vi "SaveLogEntry.vi"(8 "error in (no error)":errorcluster, 11 "Logger in":refnum<class "Logger.lvclass">) -> (0 "error out":errorcluster, 3 "Logger out":refnum<class "Logger.lvclass">)   [LabVIEW 2013, in "Logger.lvclass"]
uses:
  Logger.lvclass
  Logger.lvclass/Logger.ctl
  <vilib>/Utility/file.llb/Write To Spreadsheet File (string).vi
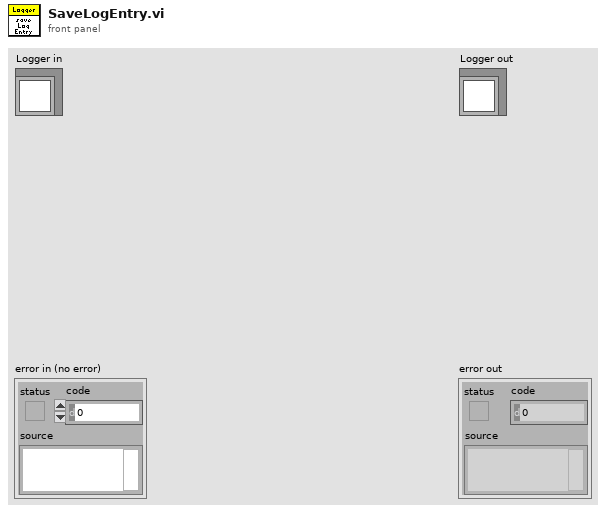
[diagram p1: front panel]
types:
  T1 = typedef "M2AADTTypedefs.lvlib/InputData.ctl" = cluster{"Limit Switches":T2, "SSI Encoder":i32, "Force Measured":T3, "Distance Data":T4, "Thermocouple Data":T5, "Stiffness Data":T6}
  T2 = typedef "ILCCommon.lvlib/ILCTypedefs.lvlib/LimitSwitches.ctl" = cluster{"1":bool, "2":bool}
  T3 = typedef "M2AADTTypedefs.lvlib/ForceDemand.ctl" = dbl[unit]
  T4 = typedef "M2AADTTypedefs.lvlib/Distance Data.ctl" = cluster{"Distance Measured 1":dbl[unit], "Distance Measured 2":dbl[unit]}
  T5 = typedef "M2AADTTypedefs.lvlib/ThermocoupleData.ctl" = cluster{"Motor Temperature":dbl[unit]}
  T6 = typedef "M2AADTTypedefs.lvlib/StiffnessData.ctl" = cluster{"Constrained Displacement":dbl[unit], "Stiffness":dbl[unit]}
  T7 = typedef "M2AADTTypedefs.lvlib/ControllerData.ctl" = cluster{"Force Demand":T3, "Force Error":T3}
  T8 = typedef "M2AADTTypedefs.lvlib/OutputData.ctl" = cluster{"Step & Direction":i16}
  T9 = typedef "M2AADTTypedefs.lvlib/StateSelector.ctl" = enum16{"EndingCycleState", "FaultState", "InteractiveMotionState", "MovingToNewForceState", "OffState", "PausingState", "StandbyState", "StoppedState"}
  T10 = typedef "M2AADTTypedefs.lvlib/TestStatus.ctl" = cluster{"activeCycle":u32, "activeProfileStep":u32}
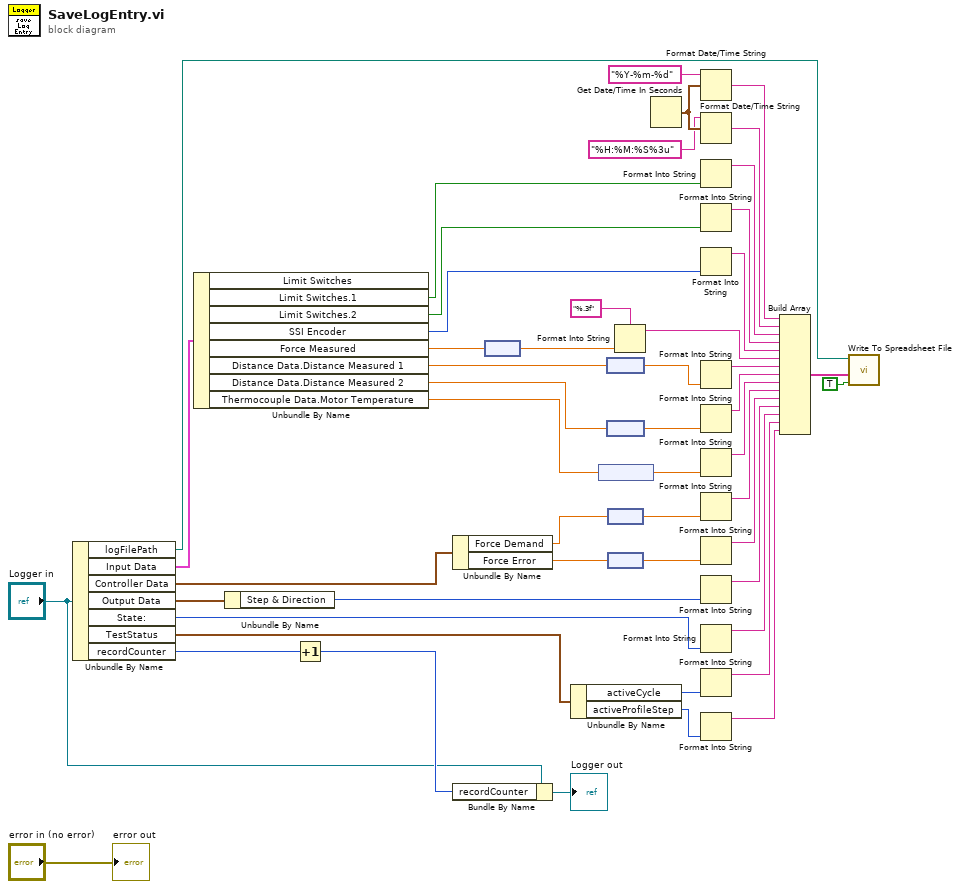
[diagram p0: block diagram]
diagram:
  n1 = Unbundle By Name("Logger in") -> ("logFilePath"=w11:path, "Input Data"=w50:T1, "Controller Data"=w48:T7, "Output Data"=w34:T8, "State:"=w31:T9, "TestStatus"=w16:T10, "recordCounter"=w10:u32)
  n2 = Unbundle By Name(w50) -> ("Limit Switches.1"=w46:bool, "Limit Switches.2"=w44:bool, "SSI Encoder"=w42:i32, "Force Measured"=w28:T3, "Distance Data.Distance Measured 1"=w26:dbl[unit], "Distance Data.Distance Measured 2"=w24:dbl[unit], "Thermocouple Data.Motor Temperature"=w22:dbl[unit])  [unwired: 1 out]
  n3 = Unbundle By Name(w34) -> ("Step & Direction"=w33:i16)
  n4 = Increment(x=w10) -> (x+1=w9:u32)
  n5 = Unbundle By Name(w48) -> ("Force Demand"=w20:T3, "Force Error"=w18:T3)
  n6 = Bundle By Name(cluster="Logger in", "recordCounter"=w9) -> (→"Logger out":refnum<class "Logger.lvclass">)
  n7 = node(w28) -> (w27:dbl)
  n8 = Unbundle By Name(w16) -> ("activeCycle"=w15:u32, "activeProfileStep"=w14:u32)
  n9 = node(w22) -> (w21:dbl)
  n10 = node(w26) -> (w25:dbl)
  n11 = node(w24) -> (w23:dbl)
  n12 = node(w20) -> (w19:dbl)
  n13 = node(w18) -> (w17:dbl)
  n14 = Format Into String(format string="%.3f", w27) -> (resulting string=w40:string)  [unwired: 2 in, 1 out]
  n15 = Get Date/Time In Seconds() -> (seconds since 1Jan1904=w6:timestamp)
  n16 = Format Date/Time String(time format string (%c)="%Y-%m-%d" ("format string"), seconds (now)=w6) -> (date/time string=w3:string)  [unwired: 1 in]
  n17 = Format Date/Time String(time format string (%c)="%H:%M:%S%3u", seconds (now)=w6) -> (date/time string=w4:string)  [unwired: 1 in]
  n18 = Format Into String(w46) -> (resulting string=w45:string)  [unwired: 3 in, 1 out]
  n19 = Format Into String(w44) -> (resulting string=w43:string)  [unwired: 3 in, 1 out]
  n20 = Format Into String(w42) -> (resulting string=w41:string)  [unwired: 3 in, 1 out]
  n21 = Format Into String(w25) -> (resulting string=w39:string)  [unwired: 3 in, 1 out]
  n22 = Format Into String(w23) -> (resulting string=w38:string)  [unwired: 3 in, 1 out]
  n23 = Format Into String(w21) -> (resulting string=w37:string)  [unwired: 3 in, 1 out]
  n24 = Format Into String(w19) -> (resulting string=w36:string)  [unwired: 3 in, 1 out]
  n25 = Format Into String(w17) -> (resulting string=w35:string)  [unwired: 3 in, 1 out]
  n26 = Format Into String(w33) -> (resulting string=w32:string)  [unwired: 3 in, 1 out]
  n27 = Format Into String(w31) -> (resulting string=w30:string)  [unwired: 3 in, 1 out]
  n28 = Format Into String(w15) -> (resulting string=w13:string)  [unwired: 3 in, 1 out]
  n29 = Format Into String(w14) -> (resulting string=w12:string)  [unwired: 3 in, 1 out]
  n30 = Build Array(w3, w4, w45, w43, w41, w40, w39, w38, w37, w36, w35, w32, w30, w13, w12) -> (w47:string[])
  n31 = call-poly <vilib>:"Write To Spreadsheet File.vi"("append to file? (new file:F)"=TRUE, "1D data"=w47, "file path (dialog if empty)"=w11) -> ()  [unwired: 5 in, 1 out]
  "error out" <- "error in (no error)"
